vi "add_2D_array_to_ItemNames.vi"(6 "2D_array":string[][](array[string]), 9 "column":i32, 10 "row":i32, 11 "ItemNames_in":string[][](array[string])) -> (3 "ItemNames_out":string[][](array[string]))   [LabVIEW 2019]
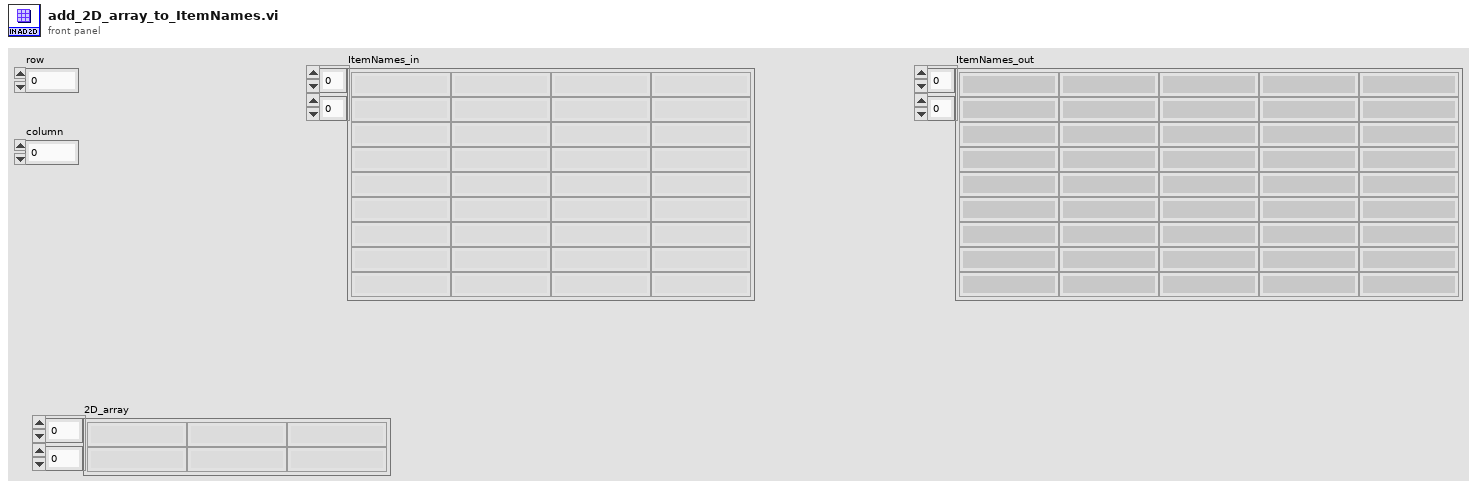
[diagram p1: front panel]
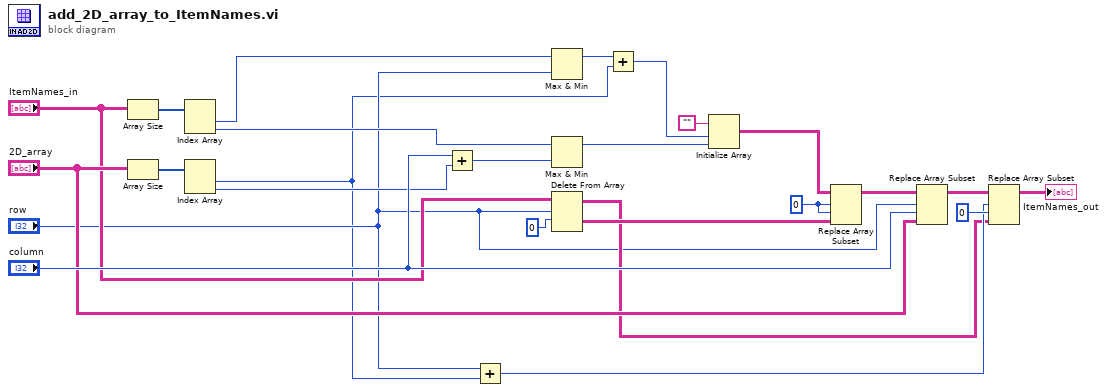
[diagram p0: block diagram]
diagram:
  w21 = 0 ("index (row)")
  n1 = Array Size(array="ItemNames_in") -> (size(s)=w24:i32[])
  n2 = Array Size(array="2D_array") -> (size(s)=w25:i32[])
  n3 = Index Array(array=w24) -> (element #1=w4:i32, element #2=w7:i32)  [unwired: 2 in]
  n4 = Index Array(array=w25) -> (element #1=w1:i32, element #2=w6:i32)  [unwired: 2 in]
  n5 = Add(x="column", y=w6) -> (x+y=w20:i32)
  n6 = Add(x="row", y=w1) -> (x+y=w13:i32)
  n7 = Max & Min(x=w4, y="row") -> (max(x,y)=w3:i32)  [unwired: 1 out]
  n8 = Max & Min(x=w7, y=w20) -> (max(x,y)=w19:i32)  [unwired: 1 out]
  n9 = Delete From Array(array="ItemNames_in", length="row", index (row)=0) -> (deleted portion=w10:string[][], array with subset deleted=w9:string[][])  [unwired: 1 in]
  n10 = Add(x=w3, y=w1) -> (x+y=w2:i32)
  n11 = Initialize Array("", w2, w19) -> (w22:string[][])
  n12 = Replace Array Subset(array=w22, new element=w10, index (row)=w21, index (col)=w21) -> (w18:string[][])
  n13 = Replace Array Subset(array=w18, new element="2D_array", index (row)="row", index (col)="column") -> (w16:string[][])
  n14 = Replace Array Subset(array=w16, new element=w9, index (row)=w13, index (col)=0 ("disabled index (col)")) -> (→"ItemNames_out":string[][])
